vi "GetPositionAndActivity.vi"(0 "handle in":i32, 1 "UnitAddress(0)":u16, 2 "MotNr(0)":u8, 3 "ResponseAddress(0)":u8, 5 "error in":errorcluster) -> (14 "handle out":i32, 15 "CurrentPosition":i32, 16 "CurrentActivity":T1, 17 "StopFlag":bool, 19 "error out":errorcluster)   [LabVIEW 2014, in "Sixpack - Driver.lvlib"]
doc: "Dieser Befehl gibt als Antwort die aktuelle Position des abgefragten Motors und Angaben über die ausgeführte Aktion zurück. Darüber hinaus gibt das STOPFLAG an, ob seit der letzten Benutzung dieses Befehls eine Stopp-Bedingung für diese Achse eingetreten ist. \n\nCMD $20\nMotorNr (0...5)\nResponseAdress: Adresse des Host zum Empfangen der Antwort Antwort\n\nAntwort\nMotorNr (0...5)\nPosAkt (signed long): aktuelle Position\nActivity: momentane Aktion (0: inaktiv, 5: Rampe, 10: PI-Regler, 15: Rotation,>= 20:Referenzfahrt\nSTOPFLAG: 1=Stop Bedingung über Schalter ist eingetreten. Wird bei Abfrage zurückgesetzt.(=0)"
uses:
  Sixpack - Driver.lvlib
  Activity.ctl
  DLL/PackDLL.dll
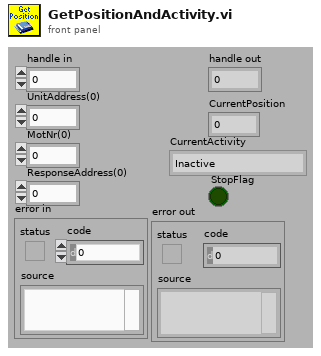
[diagram p1: front panel]
types:
  T1 = typedef "Sixpack - Driver.lvlib/Activity.ctl" = enum16{"Inactive", "Ramp", "PI-Controller", "Rotation", "ReferenceSearch", "Reference Search", "MechanicalReference"}
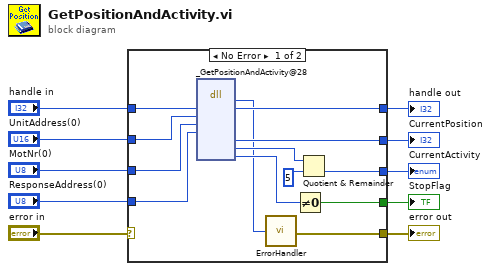
[diagram p0: block diagram]
diagram:
  n1 = case shown="No Error" "error in" {
    selector: "error in" -> [_ w24]
    tunnel: "handle in" -> [w23 w25]
    tunnel: [w22 w25] -> w9
    tunnel: "UnitAddress(0)" -> [w21 _]
    tunnel: "MotNr(0)" -> [w20 _]
    tunnel: "ResponseAddress(0)" -> [w19 _]
    tunnel: [w18 _] -> w5
    tunnel: [w15 _] -> w4
    tunnel: [w13 _] -> w3
    tunnel: [w12 w24] -> w2
    frame No Error {
      n2 = dll-call lib="D:/CS-Source/LV2014/GPL/instr.lib/SixPack/PackDLL/DLL/PackDLL.dll" fn="_GetPositionAndActivity@28" label="GetPositionAndActivity"("HANDLE"=w23, "UnitAddress"=w21, "MotNr"=w20, "ResponseAddress"=w19) -> ("BOOLEAN"=w11:i8, "HANDLE"=w22:i32, "CurrentPosition"=w18:i32, "CurrentActivity"=w16:u8, "StopFlag"=w14:u8)  [unwired: 9 in, 2 out]
      n3 = call "ErrorHandler.vi"("BOOLEAN"=w11) -> ("error out"=w12:errorcluster)
      n4 = Not Equal To 0?(x=w14) -> (x != 0?=w15:bool)
      n5 = Quotient & Remainder(x=w16, y=u8 5) -> (floor(x/y)=w13:u8)  [unwired: 1 out]
    }
    frame Error {
    }
  }
  "handle out" <- w9
  "CurrentPosition" <- w5
  "CurrentActivity" <- w3
  "StopFlag" <- w4
  "error out" <- w2
